vi "Caster.vi"(8 "error in (no error)":errorcluster, 11 "input 1":dbl) -> (0 "error out":errorcluster, 3 "String":string)   [LabVIEW 2018]
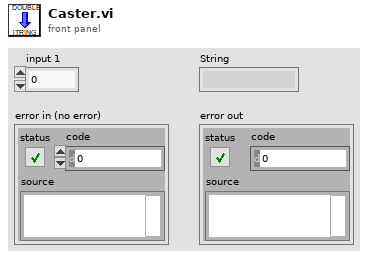
[diagram p1: front panel]
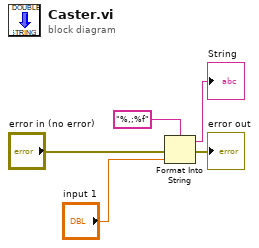
[diagram p0: block diagram]
diagram:
  n1 = Format Into String(format string="%,;%f", error in="error in (no error)", "input 1") -> (resulting string=→"String":string, error out=→"error out":errorcluster)  [unwired: 1 in]
